vi "kvCanIoCtlGet.vi"(3 "error in (no error)":errorcluster, 4 "Function":T1(ring), 5 "Channel Handle (input only)":i32) -> (0 "error out":errorcluster, 1 "Function Return Value":u32, 2 "Channel Handle (ouput only)":i32)   [LabVIEW 2022 SP3]
doc: "Performs I/O Control \"get\" functions:\n\nItem \"Get Rx Buffer Level\": returns the current RX queue level. The returned value is approximative. \n\nItem \"Get Tx Buffer Level\": returns the current TX queue level. The returned value is approximative."
uses:
  canlib32.dll
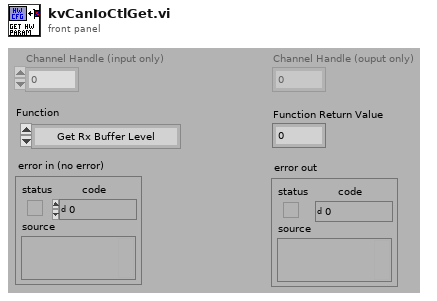
[diagram p1: front panel]
types:
  T1 = enum16{"Get Rx Buffer Level", "Get Tx Buffer Level"}
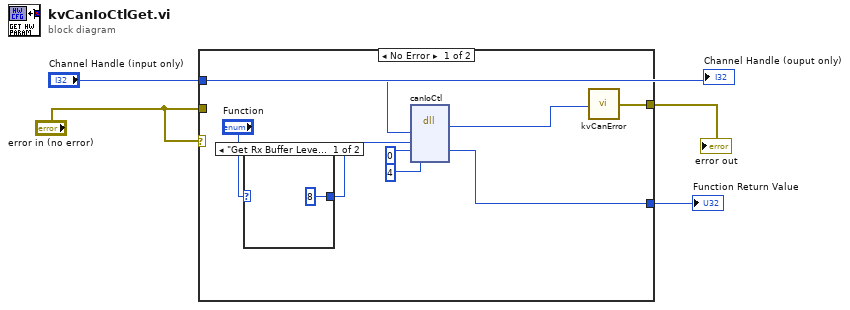
[diagram p0: block diagram]
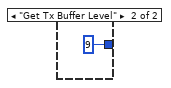
[diagram p2: hidden frame]
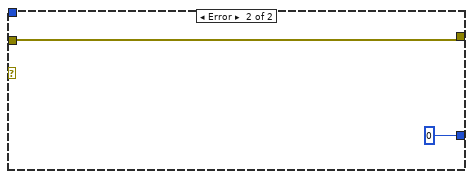
[diagram p3: hidden frame]
diagram:
  n1 = case shown="No Error" "error in (no error)" {
    tunnel: [w12 w16] -> w4
    tunnel: "error in (no error)" -> [_ w16]
    tunnel: "Channel Handle (input only)" -> [w10 _]
    tunnel: [w7 0] -> w1
    frame No Error {
      n2 = case shown="\"Get Rx Buffer Level\", Default" "Function" {
        tunnel: [8 9] -> w5
        frame "Get Rx Buffer Level", Default {
        }
        frame "Get Tx Buffer Level" {
        }
      }
      n3 = dll-call lib="canlib32.dll" fn="canIoCtl" label="Call canIoCtl"("handle"=w10, "func"=w5, "buf"=0, "buflen"=4) -> (w11:i32, "buf"=w7:u32)  [unwired: 6 in, 2 out]
      n4 = call "kvCanError.vi"("error code"=w11) -> ("error out"=w12:errorcluster)
    }
    frame Error {
    }
  }
  "error out" <- w4
  "Function Return Value" <- w1
  "Channel Handle (ouput only)" <- "Channel Handle (input only)"
